vi "Untitled 5.vi"() -> ()   [LabVIEW 2020]
uses:
  sync_type_def.ctl
panel:
  out "Element Names":string[](array[string])
  in  "sync":T1={"elyse/sync/NI6071E/delay"=1.5500000000000005, "elyse/sync/NI6071E/width"=1.0, "elyse/sync/frequency/delay"=10.0, "elyse/sync/frequency/width"=181000.0, "elyse/sync/WCM/delay:"=2177.9, "elyse/sync/WCM/width:"=10.0, "elyse/sync/modulator/delay"=2182.400000000002, "elyse/sync/modulator/width"=3.0, "elyse/sync/HF/delay"=2175.0, "elyse/sync/HF/width"=3.0, "elyse/sync/Faraday/delay"=5080.0, "elyse/sync/Faraday/width"=100.0, "elyse/sync/Oscilloscope/delay"=2175.0, "elyse/sync/Oscilloscope/width"=2.8, "elyse/sync/50Hz_20MHz/delay"=1.0, "elyse/sync/50Hz_20MHz/width"=5000.0, "elyse/sync/laser_HF/delay"=0.35, "elyse/sync/laser_HF/width"=0.35, "elyse/sync/IMAC/delay"=2176.0, "elyse/sync/IMAC/width"=100.0, "elyse/sync/laser/delay"=2008.3, "elyse/sync/laser/width"=10.0, "elyse/sync/oscilloscope1/delay"=2175.0, "elyse/sync/oscilloscope1/width"=10.0, "elyse/sync/oscilloscope2/delay"=2175.0, "elyse/sync/oscilloscope2/width"=100.0, "elyse/sync/detection1/delay"=500.0, "elyse/sync/detection1/width"=500.0, "elyse/sync/detection1/delay"=0.3, "elyse/sync/detection2/width"=10.0, "elyse/sync/machine/delay"=2175.0, "elyse/sync/machine/width"=100.0, "elyse/sync/n_selection"=4.0}
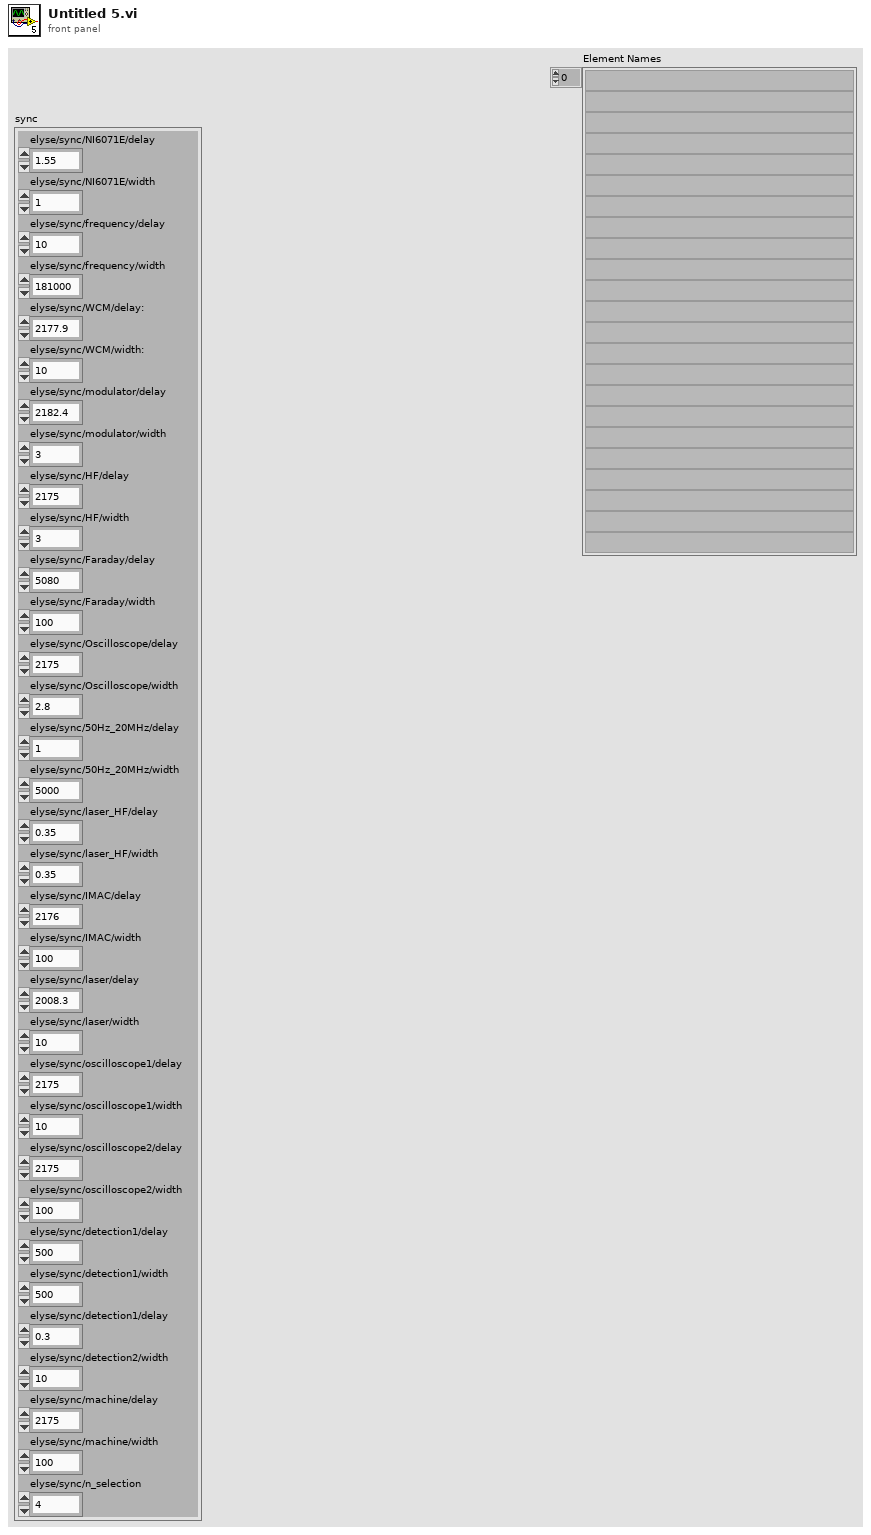
[diagram p1: front panel]
types:
  T1 = typedef "sync_type_def.ctl" = cluster{"elyse/sync/NI6071E/delay":dbl, "elyse/sync/NI6071E/width":dbl, "elyse/sync/frequency/delay":dbl, "elyse/sync/frequency/width":dbl, "elyse/sync/WCM/delay:":dbl, "elyse/sync/WCM/width:":dbl, "elyse/sync/modulator/delay":dbl, "elyse/sync/modulator/width":dbl, "elyse/sync/HF/delay":dbl, "elyse/sync/HF/width":dbl, "elyse/sync/Faraday/delay":dbl, "elyse/sync/Faraday/width":dbl, "elyse/sync/Oscilloscope/delay":dbl, "elyse/sync/Oscilloscope/width":dbl, "elyse/sync/50Hz_20MHz/delay":dbl, "elyse/sync/50Hz_20MHz/width":dbl, "elyse/sync/laser_HF/delay":dbl, "elyse/sync/laser_HF/width":dbl, "elyse/sync/IMAC/delay":dbl, "elyse/sync/IMAC/width":dbl, "elyse/sync/laser/delay":dbl, "elyse/sync/laser/width":dbl, "elyse/sync/oscilloscope1/delay":dbl, "elyse/sync/oscilloscope1/width":dbl, "elyse/sync/oscilloscope2/delay":dbl, "elyse/sync/oscilloscope2/width":dbl, "elyse/sync/detection1/delay":dbl, "elyse/sync/detection1/width":dbl, "elyse/sync/detection1/delay":dbl, "elyse/sync/detection2/width":dbl, "elyse/sync/machine/delay":dbl, "elyse/sync/machine/width":dbl, "elyse/sync/n_selection":dbl}
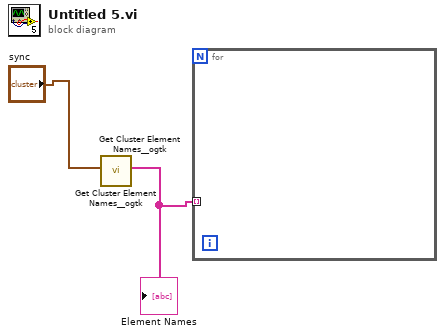
[diagram p0: block diagram]
diagram:
  n1 = call <userlib>:"Get Cluster Element Names__ogtk.vi"() -> ()  [unwired: 10 in, 2 out]
  n2 = call <userlib>:"Get Cluster Element Names__ogtk.vi"("Cluster"="sync") -> ("Element Names"=w1:string[])  [unwired: 9 in, 1 out]
  "Element Names" <- w1
  n3 = for {
    tunnel: w1 -> [_] mode=indexing
  }
